vi "TestingMATLABCalcs4T4.vi"(4 "Online":dbl[](array[numeric])=[0.0], 6 "gate_size":dbl=37.5, 7 "hitran":dbl[][](array[numeric]), 8 "lambda_off":dbl=828.45, 9 "T0_C":dbl=27.0, 10 "P0_mb":dbl=1000.0, 11 "lambda":dbl=828.195) -> (1 "sigma_off_total":dbl[](array[numeric])=[3.907720227497319e-108, 3.112137008956545e-108, 2.48353205254441e-108], 2 "sigma_on_total":dbl[](array[numeric])=[1.2232851917977358e-23, 1.218130035326043e-23, 1.2129938362952132e-23])   [LabVIEW 2012]
uses:
  <vilib>/Utility/file.llb/Read From Spreadsheet File (DBL).vi
  <vilib>/Analysis/8numeric.llb/2D Numeric Integration.vi
  <vilib>/Analysis/NI_AALPro.lvlib
panel:
  out "subarray":dbl[][](array[numeric])
  out "HitranPath":path=path "C:/Users/eol-lidar-admin/WVD-MCSupdate/WVDoldSoftware/20171016_WVDIALLabviewSlimmed/HiranData/815nm_841nm_HITRAN_2008.csv"
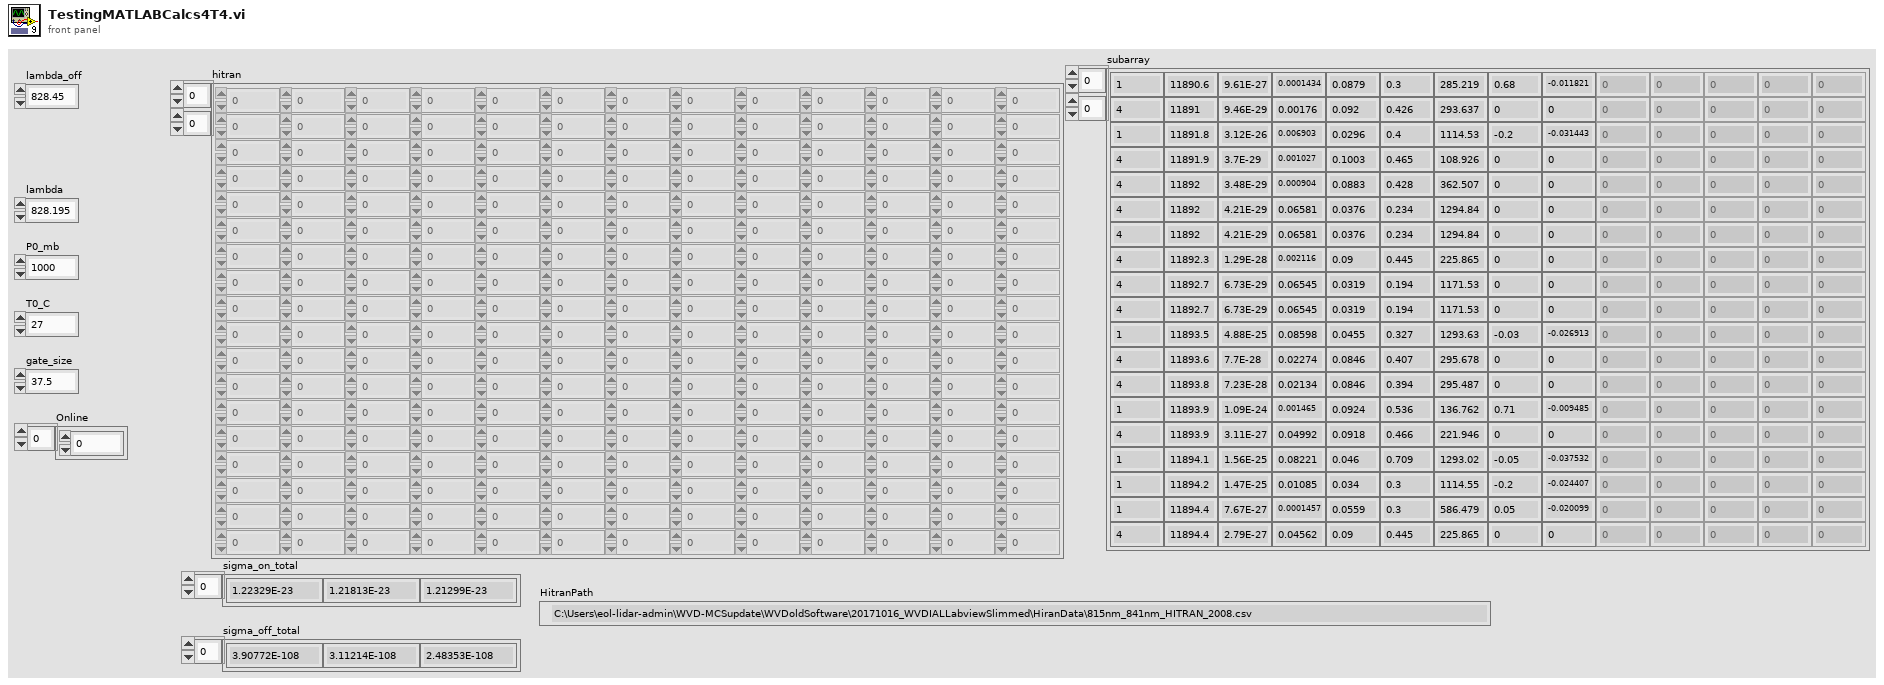
[diagram p1: front panel]
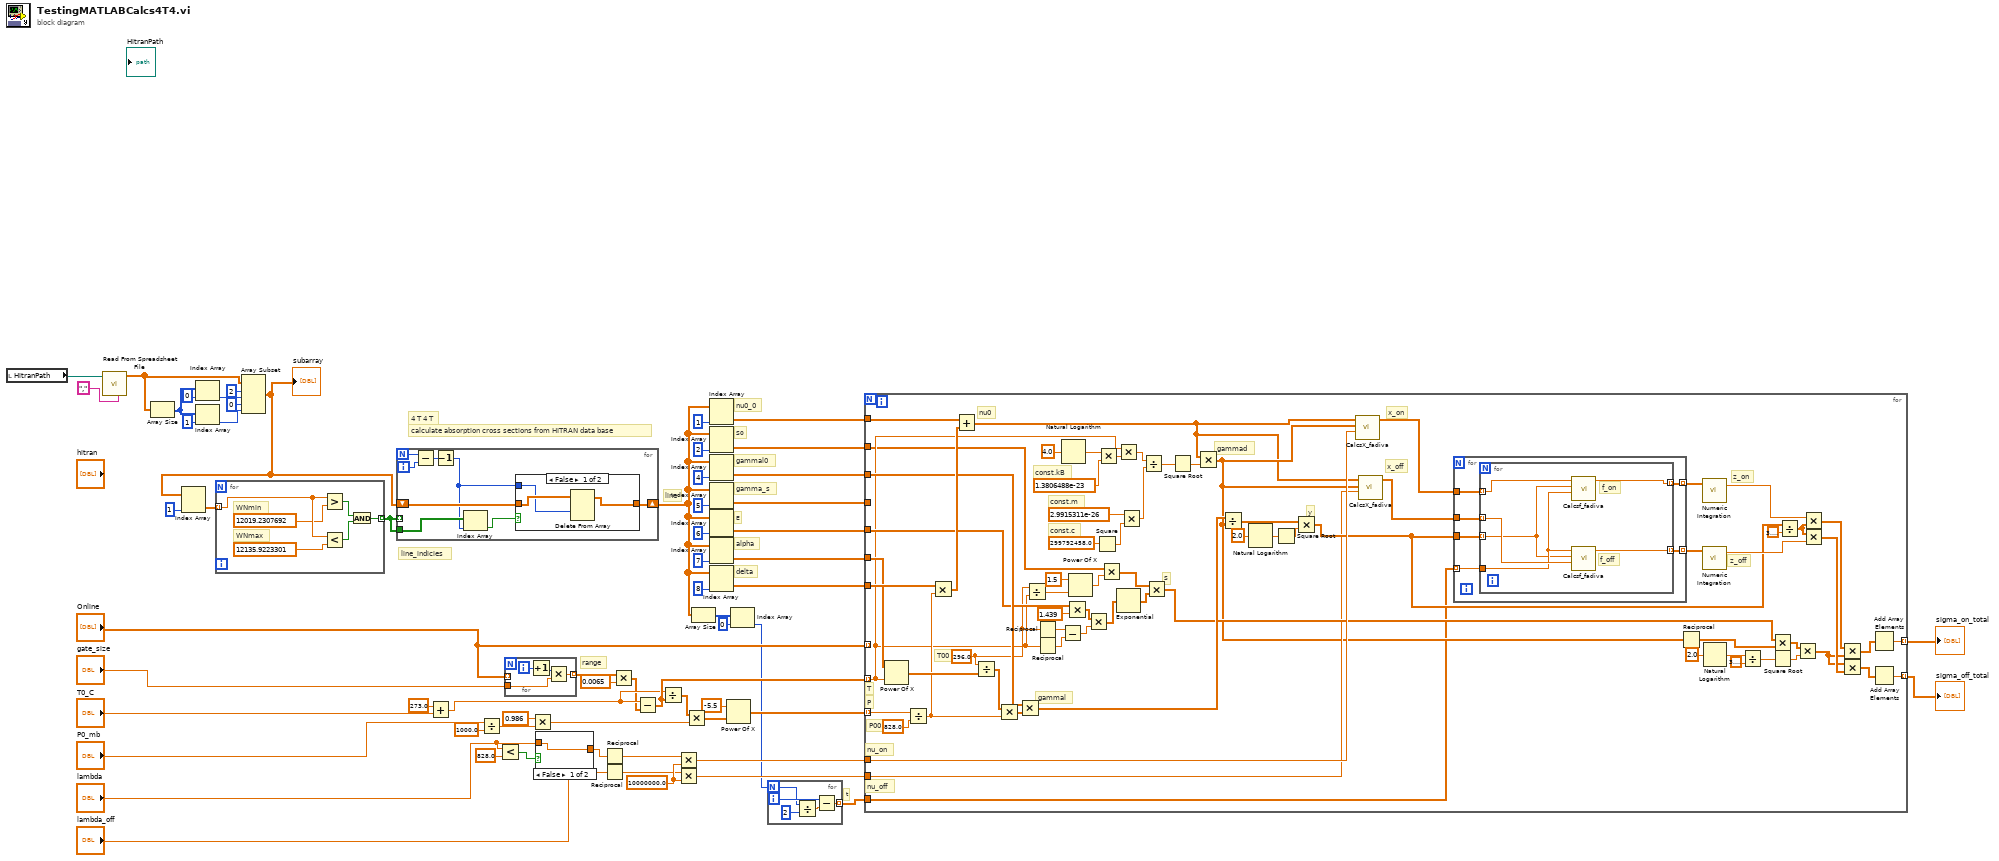
[diagram p0: block diagram]
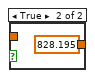
[diagram p3: hidden frame]
diagram:
  w46 = 10000000.0 ("y")
  # "t"
  # "delta"
  # "alpha"
  # "E"
  # "gamma_s"
  # "gammal0"
  # "S0"
  # "nu0_0"
  # "line"
  # "line_indicies"
  # "range"
  # "4 T 4 T"
  # "calculate absorption cross sections from HITRAN data base"
  n1 = local read "HitranPath"() -> (w2:path)
  n2 = call-poly <vilib>:"Read From Spreadsheet File.vi"("delimiter (\\t)"="," ("delimiter (\\t)"), "file path (dialog if empty)"=w2) -> ("all rows"=w3:dbl[][])  [unwired: 5 in, 4 out]
  n3 = Array Size(array=w3) -> (size(s)=w8:i32[])
  n4 = Index Array(array=w8, index=0) -> (element=w7:i32)
  n5 = Index Array(array=w8, index=1) -> (element=w6:i32)
  n6 = Array Subset(array=w3, index (row)=2 ("index"), length (row)=w7, index (col)=0 ("index"), length (col)=w6) -> (w1:dbl[][])
  "subarray" <- w1
  n7 = Index Array(array=w1, index (col)=1 ("disabled index (col)")) -> (element=w33:dbl[])  [unwired: 1 in]
  n8 = for {
    tunnel: w33 -> [w69] mode=indexing
    tunnel: [w64] -> w34 mode=indexing
    # "WNmax"
    # "WNmin"
    n9 = Greater?(x=w69, y=12019.2307692) -> (0:w65:bool)
    n10 = Less?(x=w69, y=12135.9223301) -> (x < y?=w66:bool)
    n11 = And(x=w65, y=w66) -> (x .and. y?=w64:bool)
  }
  n12 = for {
    N -> [w77]
    tunnel: w34 -> [_] mode=indexing
    shift-right: [w74] -> w61
    shift-left: w1 -> [w73]
    tunnel: w34 -> [w72]
    i -> [w76]
    n13 = Subtract(x=w77, y=w76) -> (x-y=w75:i32)
    n14 = Decrement(x=w75) -> (x-1=w70:i32)
    n15 = Index Array(array=w72, index=w70) -> (element=w71:bool)
    n16 = case shown="False" w71 {
      tunnel: [w78 w81] -> w74
      tunnel: w73 -> [w80 w81]
      tunnel: w70 -> [w79 _]
      frame False {
        n17 = Delete From Array(array=w80, index (row)=w79) -> (array with subset deleted=w78:dbl[][])  [unwired: 2 in, 1 out]
      }
      frame True {
      }
    }
  }
  n18 = Add(x=273.0, y="T0_C") -> (x+y=w27:dbl)
  n19 = Divide(x="P0_mb", y=1000.0) -> (x/y=w24:dbl)
  n20 = Less?(x="lambda", y=828.0) -> (x < y?=w17:bool)
  n21 = for {
    tunnel: "gate_size" -> [w83]
    tunnel: "Online" -> [_] mode=indexing
    tunnel: [w82] -> w21 mode=indexing
    i -> [w85]
    n22 = Increment(x=w85) -> (x+1=w84:i32)
    n23 = Multiply(x=w84, y=w83) -> (x*y=w82:dbl)
  }
  n24 = Multiply(x=0.986, y=w24) -> (x*y=w29:dbl)
  n25 = case shown="False" w17 {
    tunnel: [w86 828.195 ("lambda")] -> w47
    tunnel: "lambda" -> [w86 _]
    frame False {
    }
    frame True {
    }
  }
  n26 = Reciprocal(x=w47) -> (1/x=w44:dbl)
  n27 = Reciprocal(x="lambda_off") -> (1/x=w45:dbl)
  n28 = Multiply(x=w21, y=0.0065) -> (x*y=w22:dbl[])
  n29 = Subtract(x=w27, y=w22) -> (x-y=w58:dbl[])
  n30 = Divide(x=w27, y=w58) -> (x/y=w28:dbl[])
  n31 = Multiply(x=w44, y=w46) -> (x*y=w49:dbl)
  n32 = Multiply(x=w45, y=w46) -> (x*y=w50:dbl)
  n33 = Multiply(x=w28, y=w29) -> (x*y=w31:dbl[])
  n34 = Array Size(array=w61) -> (size(s)=w62:i32[])
  n35 = Index Array(array=w61, index (col)=1 ("disabled index (col)")) -> (element=w51:dbl[])  [unwired: 1 in]
  n36 = Index Array(array=w61, index (col)=2 ("disabled index (col)")) -> (element=w52:dbl[])  [unwired: 1 in]
  n37 = Index Array(array=w61, index (col)=4 ("disabled index (col)")) -> (element=w54:dbl[])  [unwired: 1 in]
  n38 = Index Array(array=w61, index (col)=5 ("disabled index (col)")) -> (element=w53:dbl[])  [unwired: 1 in]
  n39 = Index Array(array=w61, index (col)=6 ("disabled index (col)")) -> (element=w55:dbl[])  [unwired: 1 in]
  n40 = Index Array(array=w61, index (col)=7 ("disabled index (col)")) -> (element=w56:dbl[])  [unwired: 1 in]
  n41 = Index Array(array=w61, index (col)=8 ("disabled index (col)")) -> (element=w57:dbl[])  [unwired: 1 in]
  n42 = Power Of X(1:w31, 2:-5.5 ("y")) -> (0:w48:dbl[])
  n43 = Index Array(array=w62, index=0) -> (element=w13:i32)
  n44 = for {
    N: w13 -> [w91]
    tunnel: [w88] -> w12 mode=indexing
    i -> [w92]
    n45 = Divide(x=w91, y=2) -> (x/y=w89:dbl)
    n46 = Subtract(x=w92, y=w89) -> (x-y=w88:dbl)
  }
  n47 = for {
    tunnel: "Online" -> [_] mode=indexing
    tunnel: w48 -> [w162] mode=indexing
    tunnel: w49 -> [w137]
    tunnel: w50 -> [w97]
    tunnel: w51 -> [w163]
    tunnel: w52 -> [w106]
    tunnel: w53 -> [_]
    tunnel: w54 -> [w155]
    tunnel: w55 -> [w111]
    tunnel: w56 -> [w158]
    tunnel: w57 -> [w160]
    tunnel: w58 -> [w109] mode=indexing
    tunnel: [w136] -> w59 mode=indexing
    tunnel: [w135] -> w60 mode=indexing
    tunnel: w12 -> [w93]
    w110 = 296.0 ("y")
    # "x_on"
    # "y"
    # "x_off"
    # "z_off"
    # "z_on"
    # "S"
    # "gammad"
    # "const.c"
    # "const.m"
    # "const.kB"
    # "gammal"
    # "T00"
    # "nu0"
    # "P00"
    # "nu_off"
    # "nu_on"
    # "T"
    # "P"
    n48 = Power Of X(1:w109, 2:w158) -> (0:w157:dbl[])
    n49 = Divide(x=w162, y=828.0) -> (x/y=w156:dbl)
    n50 = Multiply(x=w160, y=w156) -> (x*y=w159:dbl[])
    n51 = Add(x=w163, y=w159) -> (x+y=w95:dbl[])
    n52 = Divide(x=w110, y=w157) -> (x/y=w120:dbl[])
    n53 = Multiply(x=w120, y=w156) -> (x*y=w154:dbl[])
    n54 = Multiply(x=w155, y=w154) -> (x*y=w140:dbl[])
    n55 = Divide(x=w110, y=w109) -> (x/y=w117:dbl)
    n56 = Reciprocal(x=w110) -> (1/x=w115:dbl)
    n57 = Reciprocal(x=w109) -> (1/x=w114:dbl)
    n58 = Subtract(x=w115, y=w114) -> (x-y=w113:dbl)
    n59 = Natural Logarithm(1:4.0 ("x")) -> (0:w150:dbl)
    n60 = Multiply(x=w111, y=1.439 ("x")) -> (x*y=w108:dbl[])
    n61 = Power Of X(1:w117, 2:1.5 ("y")) -> (0:w119:dbl)
    n62 = Multiply(x=w108, y=w113) -> (x*y=w107:dbl[])
    n63 = Square(x=299792458.0 ("y")) -> (x^2=w146:dbl)
    n64 = Multiply(x=w150, y=1.3806488e-23) -> (x*y=w152:dbl)
    n65 = Multiply(x=w106, y=w119) -> (x*y=w118:dbl[])
    n66 = Multiply(x=w109, y=w152) -> (x*y=w144:dbl)
    n67 = Exponential(1:w107) -> (0:w116:dbl[])
    n68 = Multiply(x=2.9915311e-26 ("y"), y=w146) -> (x*y=w148:dbl)
    n69 = Divide(x=w144, y=w148) -> (x/y=w143:dbl)
    n70 = Multiply(x=w118, y=w116) -> (x*y=w105:dbl[])
    n71 = Square Root(x=w143) -> (sqrt(x)=w153:dbl)
    n72 = Multiply(x=w95, y=w153) -> (x*y=w96:dbl[])
    n73 = Divide(x=w140, y=w96) -> (x/y=w139:dbl[])
    n74 = Natural Logarithm(1:2.0 ("x")) -> (0:w141:dbl)
    n75 = Square Root(x=w141) -> (sqrt(x)=w138:dbl)
    n76 = Multiply(x=w139, y=w138) -> (x*y=w99:dbl[])
    n77 = call "CalcsX_fadiva.vi"("nu"=w137, "gammad"=w96, "nu0"=w95) -> ("X_"=w102:dbl[])  [unwired: 8 in]
    n78 = call "CalcsX_fadiva.vi"("nu"=w97, "gammad"=w96, "nu0"=w95) -> ("X_"=w98:dbl[])  [unwired: 8 in]
    n79 = for {
      tunnel: w93 -> [w169] mode=indexing
      tunnel: w98 -> [w168]
      tunnel: w102 -> [w167]
      tunnel: w99 -> [w166]
      tunnel: [w165] -> w101 mode=indexing
      tunnel: [w164] -> w100 mode=indexing
      n80 = for {
        tunnel: w169 -> [w171]
        tunnel: w168 -> [w172] mode=indexing
        tunnel: w167 -> [w175] mode=indexing
        tunnel: w166 -> [w170] mode=indexing
        tunnel: [w174] -> w165 mode=indexing
        tunnel: [w173] -> w164 mode=indexing
        # "f_on"
        # "f_off"
        n81 = call "Calcsf_fadiva.vi"("X_"=w171, "y"=w170, "t"=w175) -> ("f_"=w174:dbl)  [unwired: 8 in]
        n82 = call "Calcsf_fadiva.vi"("X_"=w172, "y"=w170, "t"=w171) -> ("f_"=w173:dbl)  [unwired: 8 in]
      }
    }
    n83 = Reciprocal(x=w96) -> (1/x=w128:dbl[])
    n84 = call-poly <vilib>:"Numeric Integration.vi"("Input Array"=w101) -> ("result"=w103:dbl)  [unwired: 2 in, 1 out]
    n85 = call-poly <vilib>:"Numeric Integration.vi"("Input Array"=w100) -> ("result"=w104:dbl)  [unwired: 2 in, 1 out]
    n86 = Natural Logarithm(1:2.0 ("x")) -> (0:w133:dbl)
    n87 = Divide(x=w133, y=3.141592653589793) -> (x/y=w131:dbl)
    n88 = Multiply(x=w105, y=w128) -> (x*y=w129:dbl[])
    n89 = Square Root(x=w131) -> (sqrt(x)=w130:dbl)
    n90 = Divide(x=w99, y=3.141592653589793) -> (x/y=w124:dbl[])
    n91 = Multiply(x=w129, y=w130) -> (x*y=w94:dbl[])
    n92 = Multiply(x=w103, y=w124) -> (x*y=w123:dbl[])
    n93 = Multiply(x=w124, y=w104) -> (x*y=w122:dbl[])
    n94 = Multiply(x=w123, y=w94) -> (x*y=w127:dbl[])
    n95 = Multiply(x=w94, y=w122) -> (x*y=w126:dbl[])
    n96 = Add Array Elements(numeric array=w127) -> (sum=w136:dbl)
    n97 = Add Array Elements(numeric array=w126) -> (sum=w135:dbl)
  }
  "sigma_off_total" <- w60
  "sigma_on_total" <- w59
